vi "add_Accel.vi"(6 "Accel":T1, 7 "msg in":string) -> (3 "msg out":string)   [LabVIEW 2012]
doc: "Flattens an acceleration into a message"
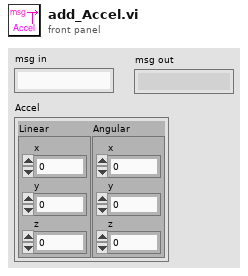
[diagram p1: front panel]
types:
  T1 = cluster{"Linear":cluster{"x":dbl, "y":dbl, "z":dbl}, "Angular":cluster{"x":dbl, "y":dbl, "z":dbl}}
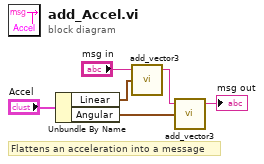
[diagram p0: block diagram]
diagram:
  # "Flattens an acceleration into a message"
  n1 = Unbundle By Name("Accel") -> ("Linear"=w2:cluster{"x":dbl, "y":dbl, "z":dbl}, "Angular"=w1:cluster{"x":dbl, "y":dbl, "z":dbl})
  n2 = call "add_vector3.vi"("Vector3"=w2, "msg in"="msg in") -> ("msg out"=w5:string)  [unwired: 3 in]
  n3 = call "add_vector3.vi"("Vector3"=w1, "msg in"=w5) -> ("msg out"=→"msg out":string)  [unwired: 3 in]
